vi "TestI2C.vi"() -> ()   [LabVIEW 2012]
uses:
  <vilib>/ni845x/ni845x.llb/ni845xControl.ctl
  <vilib>/ni845x/ni845x.llb/NI-845x Close Device Reference.vi
  <vilib>/ni845x/ni845x.llb/NI-845x I2C Close Configuration Reference.vi
  <resource>/objmgr/NI845x.rc
panel:
  in  "stop":bool
  out "Scanning":i32 format="%x"
  out "read data":u8[](array[numeric])
  out "Valid I2C":i32[](array[numeric]) format="%x"
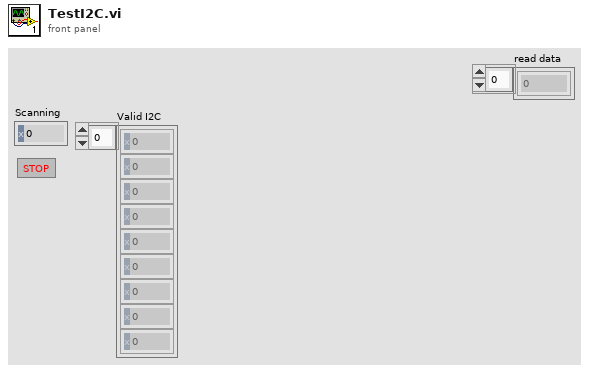
[diagram p1: front panel]
types:
  T1 = typedef "ni845xControl.ctl" = refnum<k21>
  T2 = typedef "ni845xI2cConfiguration.ctl" = refnum<k20>
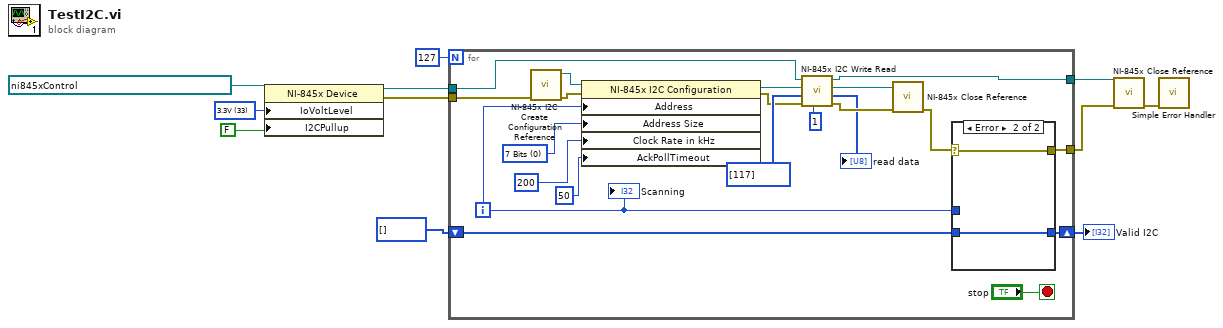
[diagram p0: block diagram]
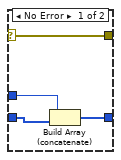
[diagram p2: hidden frame]
diagram:
  w10 = 33 items=["3.3V"=33, "2.5V"=25, "1.8V"=18, "1.5V"=15, "1.2V"=12] ("I/O Voltage Level")
  n1 = property on="Property Node" class="NI-845x Device"(reference=T1 "USB0::0x3923::0x7166::01879089::RAW" ("Device"), "IoVoltLevel"=w10, "I2CPullup"=FALSE ("I²C Pullup Enable")) -> (reference out=w2:T1, error out=w7:errorcluster)  [unwired: 1 in]
  n2 = for {
    N: 127 -> [_]
    tunnel: w7 -> [w32]
    shift-right: [w25] -> w5
    shift-left: i32[] [] ("appended array") -> [w24]
    tunnel: [w23] -> w4
    tunnel: w2 -> [w22]
    tunnel: [w14] -> w1
    i -> [w26]
    stop <- "stop" stop-if-true
    w29 = 0 items=["7 Bits", "10 Bits"] ("Address Size")
    n3 = call <vilib>:"NI-845x I2C Create Configuration Reference.vi"("error in (no error)"=w32) -> ("error out"=w30:errorcluster, "i2c configuration"=w31:T2)  [unwired: 9 out]
    n4 = property class="NI-845x I2C Configuration"(reference=w31, error in=w30, "Address"=w26, "Address Size"=w29, "Clock Rate in kHz"=u16 200, "AckPollTimeout"=u16 50 ("ACK Poll Timeout")) -> (reference out=w21:T2, error out=w18:errorcluster)
    n5 = call <vilib>:"NI-845x I2C Write Read.vi"("num bytes to read"=u32 1, "error in (no error)"=w18, "write data"=u8[] [117], "i2c configuration in"=w21, "device reference in"=w22) -> ("error out"=w16:errorcluster, "read data"=→"read data":u8[], "i2c configuration out"=w17:T2, "device reference out"=w14:T1)  [unwired: 3 in]
    n6 = call-poly <vilib>:"NI-845x Close Reference.vi"("error in (no error)"=w16, "i2c configuration"=w17) -> ("error out"=w27:errorcluster)  [unwired: 9 in]
    n7 = case shown="Error" w27 {
      selector: w27 -> [w33 w37]
      tunnel: w26 -> [w36 _]
      tunnel: [w35 w38] -> w25
      tunnel: w24 -> [w34 w38]
      tunnel: [w33 w37] -> w23
      frame No Error {
        n8 = Build Array (concatenate)(w36, w34) -> (w35:i32[])
      }
      frame Error {
      }
    }
    "Scanning" <- w26
  }
  "Valid I2C" <- w5
  n9 = call-poly <vilib>:"NI-845x Close Reference.vi"("error in (no error)"=w4, "device reference"=w1) -> ("error out"=w3:errorcluster)  [unwired: 9 in]
  n10 = call <vilib>:"Simple Error Handler.vi"("error in (no error)"=w3) -> ()  [unwired: 4 in, 5 out]
